vi "Close.vi"(8 "error in (no error)":errorcluster {"code" format="%.0x"}, 11 "VISA Resource Name":refnum<visa-resource-name>) -> (0 "error out":errorcluster {"code" format="%.0x"})   [LabVIEW 2011, in "Agilent 546XX Series.lvlib"]
doc: "This VI performs the following operations:\n\n- Closes the instrument I/O session.\n\n- Destroys the instrument driver session and all of its properties.\n\n- Deallocates any memory resources the driver uses.\n\nNotes:\n\n(1) You must unlock the session before calling ag546xx Close.\n\n(2) After calling ag546xx Close, you cannot use the instrument driver again until you call ag546xx Initialize or ag546xx Initialize With Options."
uses:
  Agilent 546XX Series.lvlib
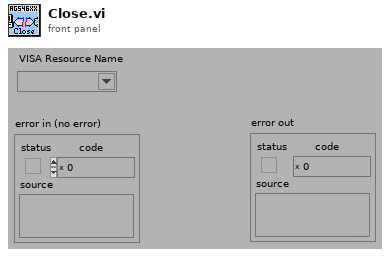
[diagram p1: front panel]
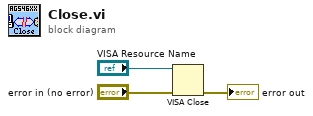
[diagram p0: block diagram]
diagram:
  n1 = VISA Close(VISA resource name="VISA Resource Name", error in (no error)="error in (no error)") -> (error out=→"error out":errorcluster)
